vi "find matching string in the list.vi"(6 "quote specials":bool, 10 "regular expression":string="aaa bbb.ccc", 11 "strings":string[](array[string])=["aaa", "bbb", "aaa bbb.ccc", "aaa bbb ccc", "dddd"]) -> (1 "match found":bool, 2 "matching string index":i32, 3 "matching string":string)   [LabVIEW 2015]
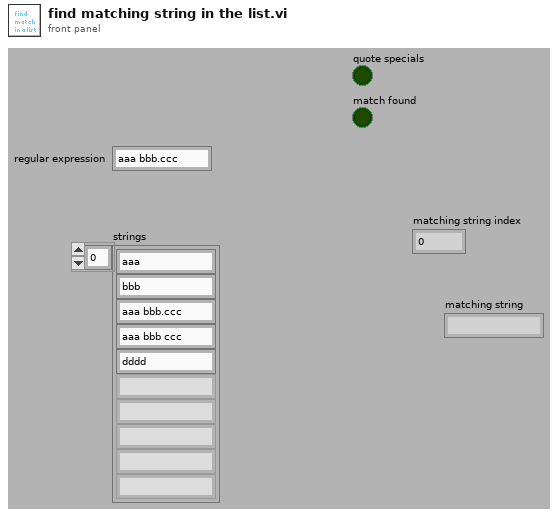
[diagram p1: front panel]
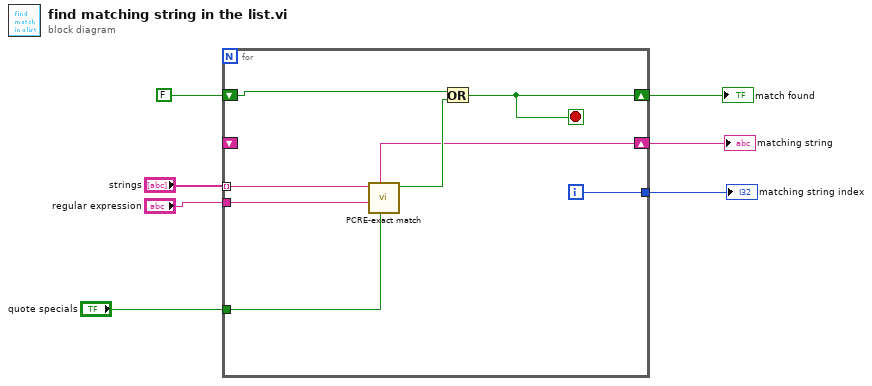
[diagram p0: block diagram]
diagram:
  n1 = for {
    tunnel: "strings" -> [w15] mode=indexing
    tunnel: "regular expression" -> [w14]
    shift-right: [w12] -> w5
    shift-left: _ -> [_]
    shift-right: [w11] -> w4
    shift-left: FALSE -> [w10]
    tunnel: [w9] -> w2
    tunnel: "quote specials" -> [w8]
    i -> [w9]
    stop <- w11 stop-if-true
    n2 = call "PCRE-exact match.vi"("quote specials"=w8, "regular expression"=w14, "input string"=w15) -> ("exact match"=w13:bool, "output string"=w12:string)  [unwired: 6 in, 1 out]
    n3 = Or(x=w10, y=w13) -> (x .or. y?=w11:bool)
  }
  "matching string" <- w5
  "match found" <- w4
  "matching string index" <- w2
